vi "Main_SERVO.vi"() -> ()   [LabVIEW 2014]
uses:
  <vilib>/myRIO/Instrument Drivers/Utilities/Utilities.lvlib
  <vilib>/myRIO/Express VI/Onboard IO/PWM/PWM Express VI.xnode
  <vilib>/myRIO/Instrument Drivers/Onboard IO/PWM/vis/Set Duty Cycle and Frequency.vi
  <vilib>/myRIO/Instrument Drivers/Onboard IO/PWM/PWM.lvlib
  <vilib>/myRIO/Instrument Drivers/Onboard IO/PWM/typedefs/PWM Configuration.ctl
  <vilib>/myRIO/Common/Instrument Driver Framework/myRIO v1.0/PWM/typedefs/PWM Channels Enum.ctl
  <vilib>/myRIO/Common/Instrument Driver Framework/Utilities/typedefs/Generic FPGA Reference.ctl
  <vilib>/myRIO/Common/Instrument Driver Framework/Utilities/typedefs/myRIO v1.0 Reference.ctl
  <vilib>/myRIO/Common/Instrument Driver Framework/Utilities/typedefs/Hardware Version Enum.ctl
  <vilib>/myRIO/Common/Instrument Driver Framework/Utilities/typedefs/myRIO Generic Hardware Reference.ctl
  <vilib>/myRIO/Instrument Drivers/Onboard IO/PWM/typedefs/PWM Reference.ctl
  <vilib>/myRIO/Instrument Drivers/Onboard IO/PWM/vis/myRIO PWM Open.xnode
  <vilib>/myRIO/Common/Instrument Driver Framework/Utilities/vis/Is FPGA Ref Available.vi
  <vilib>/myRIO/Common/Instrument Driver Framework/myRIO v1.0/PWM/vis/myRIO v1.1 Open PWM.vi
  <vilib>/userdefined/High Color/nirio_resource_hc.ctl
panel:
  in  "Knob":dbl(knob)=1.5 scale=0.8..2.2 scale format="%#_3g"
  in  "Knob 2":dbl(knob)=1.5 scale=0.8..2.2 scale format="%#_3g"
  in  "Knob 3":dbl(knob)=1.5 scale=0.8..2.2 scale format="%#_3g"
  in  "[ESC]":bool
  # "Servo Testing"
  # "Pulse Width (ms)"
  # "Pulse Width (ms)"
  # "Pulse Width (ms)"
  # "SERVO 0"
  # "SERVO 1"
  # "SERVO 2"
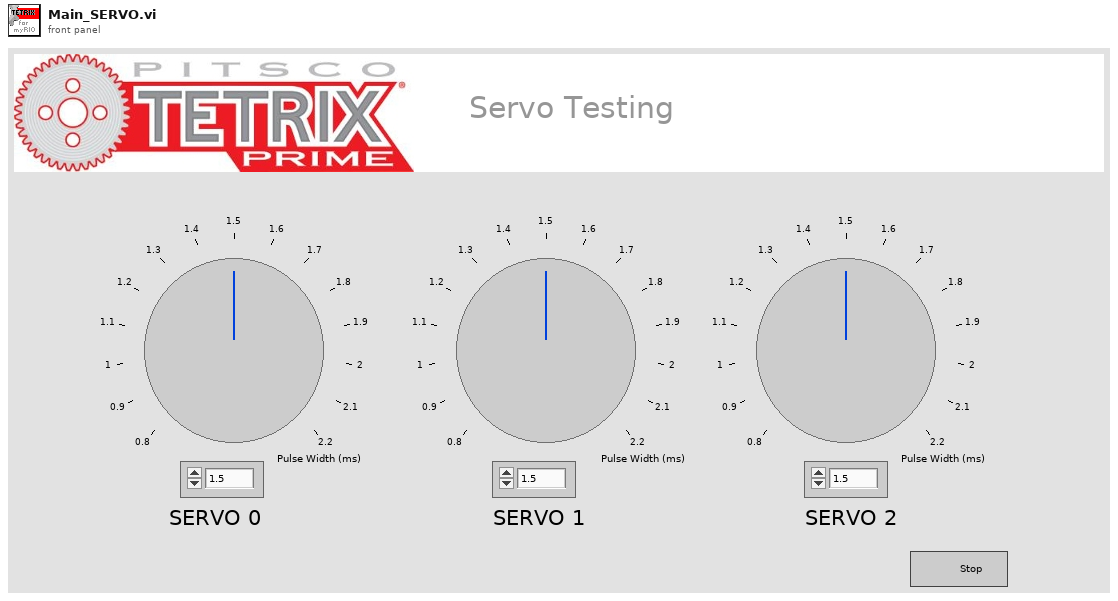
[diagram p1: front panel]
types:
  T1 = typedef "PWM.lvlib/PWM Reference.ctl" = cluster{"myRIO Reference":T2, "PWM Channels Enum":T6, "PWM Configuration":T7}
  T2 = typedef "myRIO Generic Hardware Reference.ctl" = cluster{"myRIO Model":T3, "myRIO Hardware Reference":T4}
  T3 = typedef "Hardware Version Enum.ctl" = enum16{"Unknown", "myRIO-1900", "myRIO-1950"}
  T4 = typedef "myRIO v1.0 Reference.ctl" = cluster{"Generic FPGA Reference":T5, "Allow multiple opens":bool}
  T5 = typedef "Generic FPGA Reference.ctl" = refnum<k20>
  T6 = typedef "PWM Channels Enum.ctl" = enum16{"Not Connected", "C/PWM0", "C/PWM1", "A/PWM0", "A/PWM1", "A/PWM2", "B/PWM0", "B/PWM1", "B/PWM2"}
  T7 = typedef "PWM.lvlib/PWM Configuration.ctl" = cluster{"Frequency":dbl, "Duty Cycle":dbl}
  T8 = typedef "nirio_resource_hc.ctl" = tag
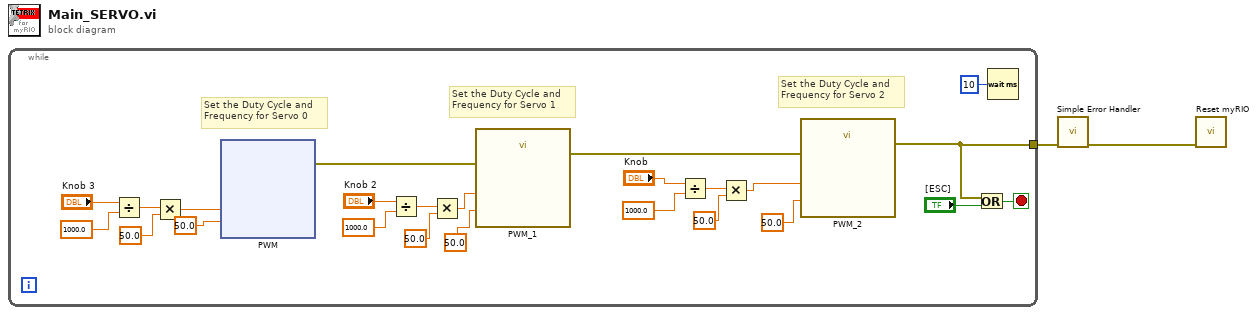
[diagram p0: block diagram]
diagram:
  n1 = while {
    tunnel: [w21] -> w1
    stop <- w26 stop-if-true
    # "Set the Duty Cycle and \nFrequency for Servo 2"
    # "Set the Duty Cycle and \nFrequency for Servo 1"
    # "Set the Duty Cycle and \nFrequency for Servo 0"
    n2 = Divide(x="Knob 3", y=1000.0) -> (x/y=w15:dbl)
    n3 = Multiply(x=w15, y=50.0) -> (x*y=w13:dbl)
    n4 = xnode "PWM"("Duty Cycle"=w13, "Frequency [Hz]"=50.0 ("Frequency (Hz)")) -> ("error out"=w23:errorcluster)  [unwired: 1 in]
    n5 = Divide(x="Knob 2", y=1000.0) -> (x/y=w11:dbl)
    n6 = Multiply(x=w11, y=50.0) -> (x*y=w5:dbl)
    n7 = call "PWM_1"("Duty Cycle (0-1)"=w5, "Frequency (Hz)"=50.0, "error in (no error)"=w23) -> ("error out"=w22:errorcluster)  [unwired: 24 in]
    n8 = Divide(x="Knob", y=1000.0) -> (x/y=w8:dbl)
    n9 = Multiply(x=w8, y=50.0) -> (x*y=w3:dbl)
    n10 = call "PWM_2"("Duty Cycle (0-1)"=w3, "Frequency (Hz)"=50.0, "error in (no error)"=w22) -> ("error out"=w21:errorcluster)  [unwired: 24 in]
    n11 = Or(x=w21, y="[ESC]") -> (x .or. y?=w26:bool)
    n12 = Wait (ms)(milliseconds to wait=u32 10) -> ()  [unwired: 1 out]
  }
  n13 = call <vilib>:"Simple Error Handler.vi"("error in (no error)"=w1) -> ("error out"=w2:errorcluster)  [unwired: 4 in, 4 out]
  n14 = call <vilib>:"Reset myRIO.vi"("error in (no error)"=w2) -> ()  [unwired: 10 in, 1 out]
